vi "Correct_Position_info.vi"() -> (0 "error out":errorcluster, 4 "Path":path)   [LabVIEW 2011]
panel:
  out "File Changed":bool
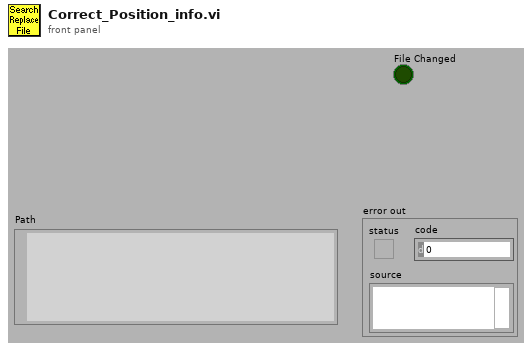
[diagram p1: front panel]
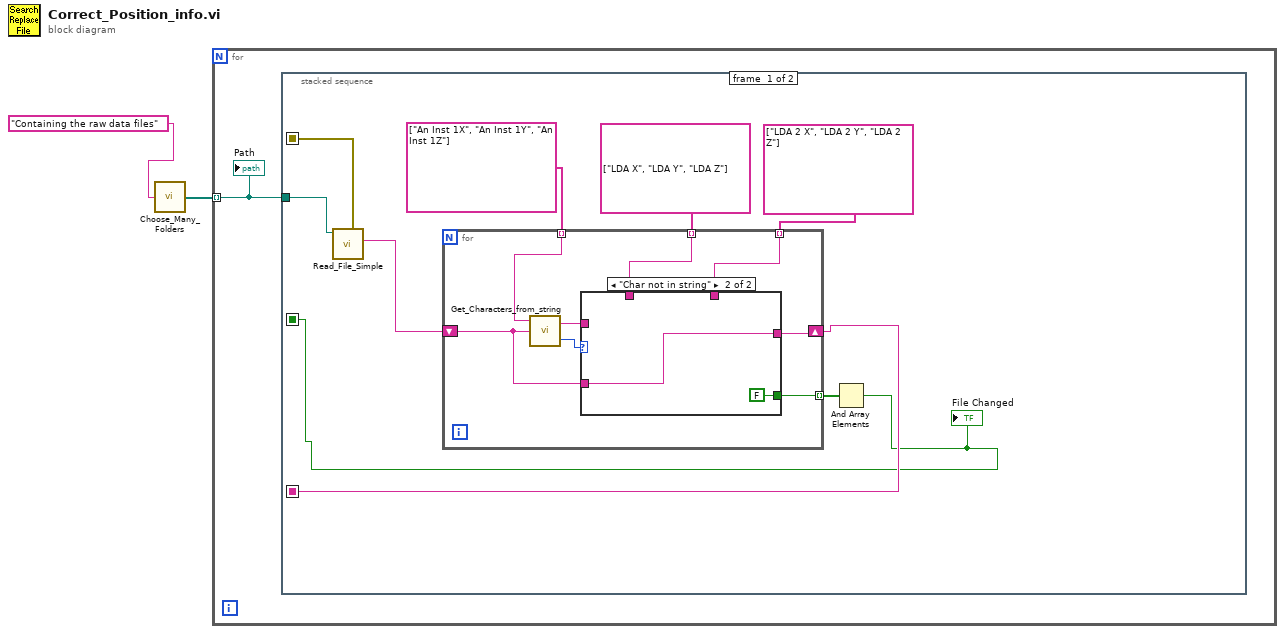
[diagram p0: block diagram]
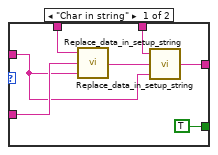
[diagram p2: hidden frame]
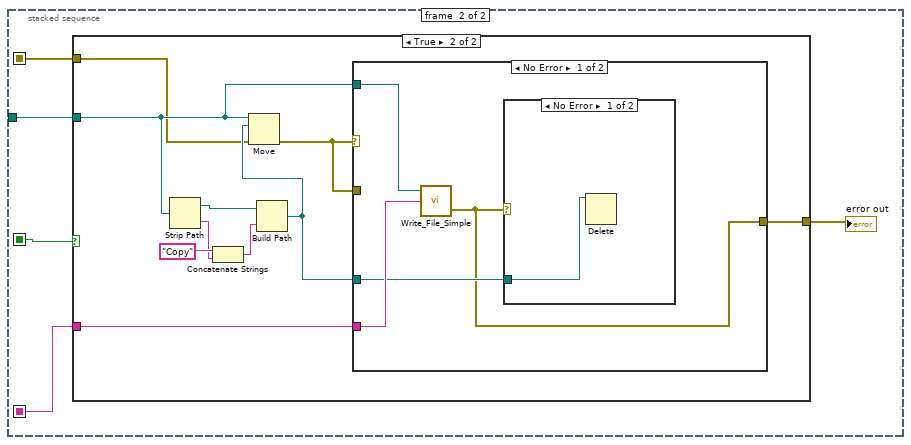
[diagram p3: hidden frame]
diagram:
  n1 = call "Choose_Many_Folders.vi"("Purpose of choosing folder"="Containing the raw data files") -> ("Files"=w1:path[])
  n2 = for {
    tunnel: w1 -> [w3] mode=indexing
    n3 = stacked-sequence {
      seq-local: [w11 _] -> [_ w30]
      seq-local: [w8 _] -> [_ w32]
      seq-local: [w4 _] -> [_ w31]
      tunnel: w3 -> [w12 w34]
      frame #0 {
        n4 = call "Read_File_Simple.vi"("Filename"=w12) -> ("error out"=w11:errorcluster, "string"=w7:string)  [unwired: 4 in, 4 out]
        n5 = for {
          shift-right: [w16] -> w8
          shift-left: w7 -> [w17]
          tunnel: string[] ["An Inst 1X", "An Inst 1Y", "An Inst 1Z"] -> [w20] mode=indexing
          tunnel: string[] ["LDA X", "LDA Y", "LDA Z"] -> [w19] mode=indexing
          tunnel: string[] ["LDA 2 X", "LDA 2 Y", "LDA 2 Z"] -> [w18] mode=indexing
          tunnel: [w13] -> w5 mode=indexing
          n6 = call "Get_Characters_from_string.vi"("Input string"=w17, "Variable name"=w20) -> ("Status"=w14:enum16{"Char in string", "Char not in string"}, "Value"=w15:string)  [unwired: 1 in]
          n7 = case shown="\"Char not in string\"" w14 {
            tunnel: w19 -> [w27 _]
            tunnel: w18 -> [w26 _]
            tunnel: w17 -> [w25 w29]
            tunnel: [w24 w29] -> w16
            tunnel: w15 -> [w22 _]
            tunnel: [TRUE FALSE] -> w13
            frame "Char in string" {
              n8 = call "Replace_data_in_setup_string.vi"("New data string"=w22, "Input string"=w25, "Variable name"=w27) -> ("Appended string"=w23:string)
              n9 = call "Replace_data_in_setup_string.vi"("New data string"=w22, "Input string"=w23, "Variable name"=w26) -> ("Appended string"=w24:string)
            }
            frame "Char not in string" {
            }
          }
        }
        n10 = And Array Elements(Boolean array=w5) -> (logical AND=w4:bool)
        "File Changed" <- w4
      }
      frame #1 {
        n11 = case shown="True" w31 {
          tunnel: w34 -> [_ w41]
          tunnel: w32 -> [_ w40]
          tunnel: [w35 w38] -> w33
          tunnel: w30 -> [w35 w36]
          frame False {
          }
          frame True {
            n12 = Strip Path(path=w41) -> (stripped path=w42:path, name=w44:string)
            n13 = Concatenate Strings("Copy" ("name or relative path"), w44) -> (w43:string)
            n14 = Build Path(base path=w42, name or relative path=w43) -> (appended path=w39:path)
            n15 = Move(source path=w41, error in=w36, 10:w39) -> (error out=w37:errorcluster)  [unwired: 2 in, 2 out]
            n16 = case shown="No Error" w37 {
              tunnel: w41 -> [w49 _]
              tunnel: w40 -> [w48 _]
              tunnel: w39 -> [w47 _]
              tunnel: [w46 w51] -> w38
              tunnel: w37 -> [_ w51]
              frame No Error {
                n17 = call "Write_File_Simple.vi"("character string"=w48, "file path"=w49) -> ("error out"=w46:errorcluster)  [unwired: 1 in, 1 out]
                n18 = case shown="No Error" w46 {
                  tunnel: w47 -> [w50 _]
                  frame No Error {
                    n19 = Delete(path (use dialog)=w50) -> ()  [unwired: 4 in, 3 out]
                  }
                  frame Error {
                  }
                }
              }
              frame Error {
              }
            }
          }
        }
        "error out" <- w33
      }
    }
    "Path" <- w3
  }
